vi "Read On Timeout Status.vi"(8 "error in (no error)":errorcluster, 11 "Repeat Until Timeout in":refnum<class "Repeat Until Timeout.lvclass">) -> (0 "error out":errorcluster, 2 "On Count Status":T1, 3 "Repeat Until Timeout out":refnum<class "Repeat Until Timeout.lvclass">)   [LabVIEW 2021, in "BT.lvlib" / "Repeat Until Timeout.lvclass"]
uses:
  Repeat Until Timeout.lvclass
  Support/On Timeout Status - Type.ctl
  Repeat Until Timeout.lvclass/Repeat Until Timeout.ctl
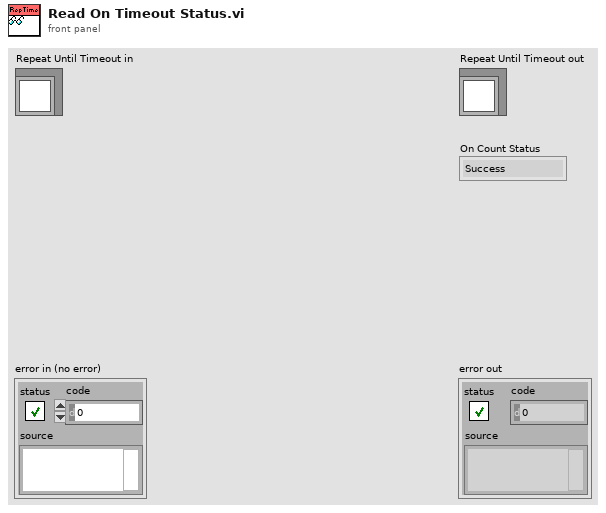
[diagram p1: front panel]
types:
  T1 = typedef "BT.lvlib/Repeat Until Timeout.lvclass/On Timeout Status - Type.ctl" = enum16{"Success", "Failure"}
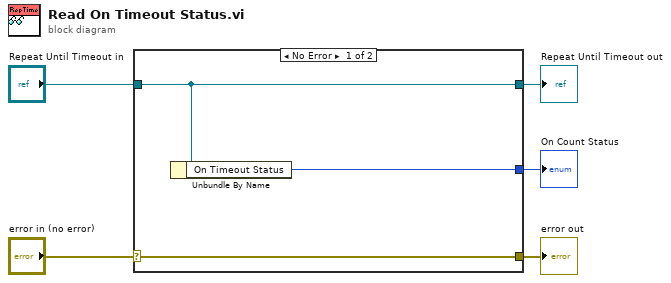
[diagram p0: block diagram]
diagram:
  n1 = case shown="No Error" "error in (no error)" {
    selector: "error in (no error)" -> [w8 w9]
    tunnel: [w8 w9] -> w4
    tunnel: [w7 w10] -> w2
    tunnel: "Repeat Until Timeout in" -> [w7 w10]
    tunnel: [w6 _] -> w1
    frame No Error {
      n2 = Unbundle By Name(w7) -> ("On Timeout Status"=w6:T1)
    }
    frame Error {
    }
  }
  "error out" <- w4
  "Repeat Until Timeout out" <- w2
  "On Count Status" <- w1
